vi "Stop Device.vi"(8 "error in":errorcluster, 11 "TE Cooler in":refnum<class "TE Cooler.lvclass">) -> (0 "error out":errorcluster, 3 "TE Cooler out":refnum<class "TE Cooler.lvclass">)   [LabVIEW 2015, in "TE Cooler.lvlib" / "TE Cooler.lvclass"]
uses:
  TE Cooler.lvclass
  TE Cooler.lvclass/TE Cooler.ctl
  reusable/Session APIs/Serial/Serial Session.lvclass
  Generic TEC/TEC.lvclass
  <vilib>/MSR Consulting, LLC/ESF/Session - Root.lvclass
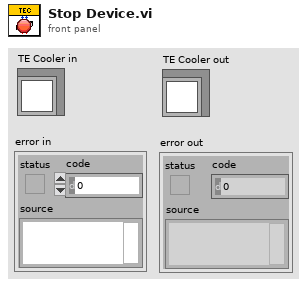
[diagram p1: front panel]
types:
  T1 = typedef "Session - Root.lvclass/Session Handle.ctl" = refnum<data-value>
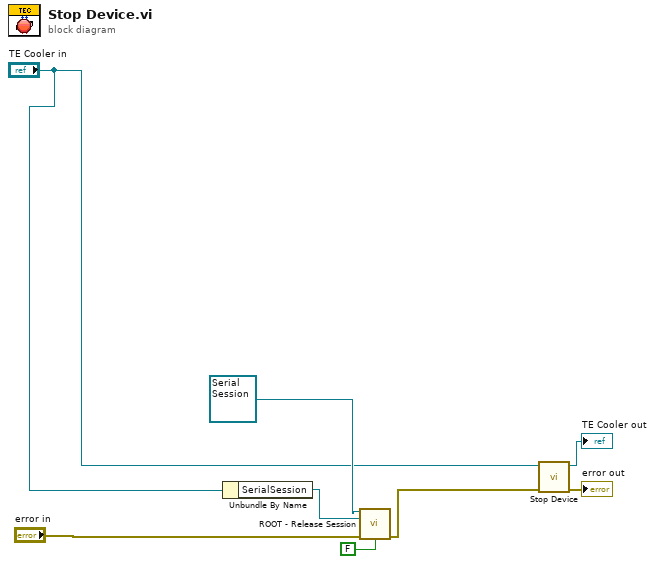
[diagram p0: block diagram]
diagram:
  n1 = Unbundle By Name("TE Cooler in") -> ("SerialSession"=w6:T1)
  n2 = call <vilib>:"ROOT - Release Session.vi"("OBJ - Session in"=refnum<class "Serial Session.lvclass"> refnum ("Serial Session"), "Session Handle in"=w6, "error in (no error)"="error in", "force destroy? (F)"=FALSE) -> ("error out"=w1:errorcluster)  [unwired: 10 in, 1 out]
  n3 = call-parent "Stop Device.vi"("error in"=w1, "Configurable Device in"="TE Cooler in") -> ("error out"=→"error out":errorcluster, "Configurable Device out"=→"TE Cooler out":refnum<class "TE Cooler.lvclass">)  [unwired: 8 in]
